vi "test_ParseSolutionFile.vi"() -> (3 "Pass?":bool)   [LabVIEW 2020, in "Tests.SolutionBuilder.lvlib"]
uses:
  Tests.SolutionBuilder.lvlib
  SolutionBuilder/SolutionBuilder.lvclass
panel:
  out "test results":u32 format="%03b"
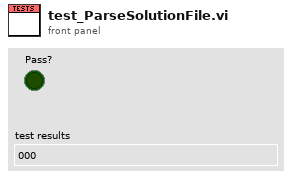
[diagram p1: front panel]
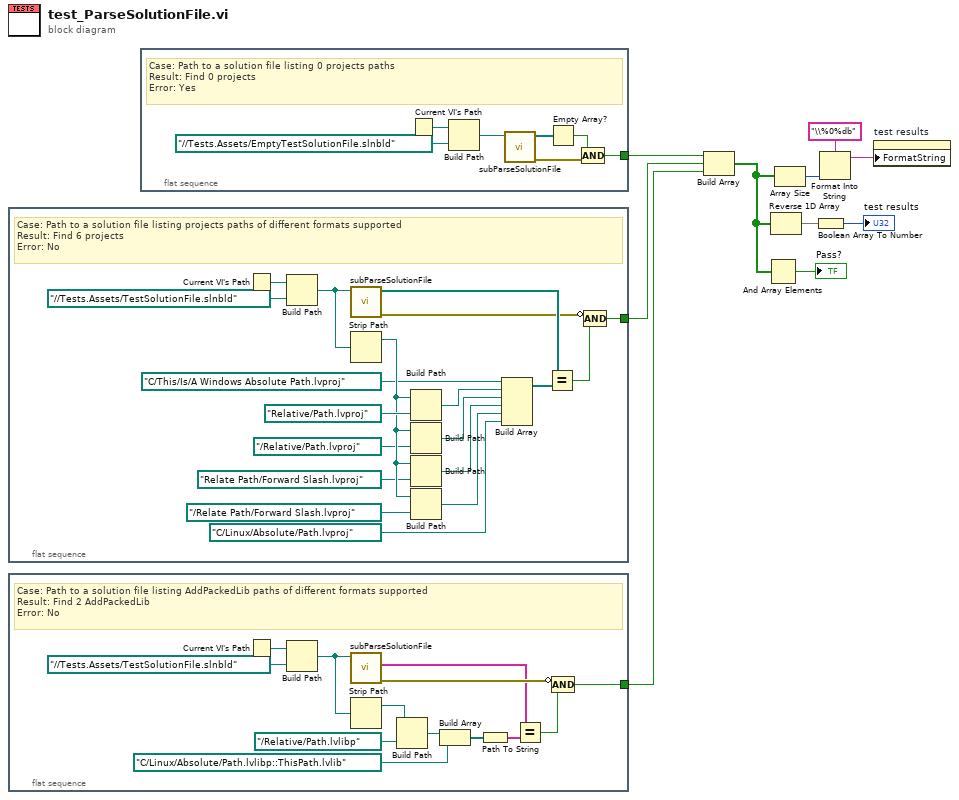
[diagram p0: block diagram]
diagram:
  n1 = flat-sequence {
    tunnel: [w11] -> w4
    frame #0 {
      # "Case: Path to a solution file listing projects paths of different formats supported\nResult: Find 6 projects\nError: No"
      n2 = Current VI's Path() -> (path=w29:path)
      n3 = Build Path(base path=w29, name or relative path=path "../../Tests.Assets/TestSolutionFile.slnbld" ("Path")) -> (appended path=w15:path)
      n4 = call "subParseSolutionFile.vi"("Solution file"=w15) -> ("error out"=w13:errorcluster, "Projects"=w14:path[])  [unwired: 8 in, 1 out]
      n5 = Strip Path(path=w15) -> (stripped path=w26:path)  [unwired: 1 out]
      n6 = Build Path(base path=w26, name or relative path=path "Relative/Path.lvproj" ("Path")) -> (appended path=w21:path)
      n7 = Build Path(base path=w26, name or relative path=path "../Relative/Path.lvproj" ("Path")) -> (appended path=w20:path)
      n8 = Build Path(base path=w26, name or relative path=path "Relate Path/Forward Slash.lvproj" ("Path")) -> (appended path=w19:path)
      n9 = Build Path(base path=w26, name or relative path=path "../Relate Path/Forward Slash.lvproj" ("Path")) -> (appended path=w18:path)
      n10 = Build Array(path "C:/This/Is/A Windows Absolute Path.lvproj" ("Path"), w21, w20, w19, w18, path "C:/Linux/Absolute/Path.lvproj" ("Path")) -> (w16:path[])
      n11 = Equal?(x=w14, y=w16) -> (x = y?=w12:bool)
      n12 = Compound Arithmetic op=AND(invert w13, w12) -> (w11:bool)
    }
  }
  n13 = flat-sequence {
    tunnel: [w33] -> w2
    frame #0 {
      # "Case: Path to a solution file listing AddPackedLib paths of different formats supported\nResult: Find 2 AddPackedLib\nError: No"
      n14 = Current VI's Path() -> (path=w42:path)
      n15 = Build Path(base path=w42, name or relative path=path "../../Tests.Assets/TestSolutionFile.slnbld" ("Path")) -> (appended path=w36:path)
      n16 = call "subParseSolutionFile.vi"("Solution file"=w36) -> ("error out"=w35:errorcluster, "Lib definition strings"=w32:string[])  [unwired: 8 in, 1 out]
      n17 = Strip Path(path=w36) -> (stripped path=w39:path)  [unwired: 1 out]
      n18 = Build Path(base path=w39, name or relative path=path "../Relative/Path.lvlibp" ("Path")) -> (appended path=w38:path)
      n19 = Build Array(w38, path "C:/Linux/Absolute/Path.lvlibp::ThisPath.lvlib" ("Path")) -> (w37:path[])
      n20 = Path To String(path=w37) -> (string=w31:string[])
      n21 = Equal?(x=w32, y=w31) -> (x = y?=w34:bool)
      n22 = Compound Arithmetic op=AND(invert w35, w34) -> (w33:bool)
    }
  }
  n23 = flat-sequence {
    tunnel: [w46] -> w3
    frame #0 {
      # "Case: Path to a solution file listing 0 projects paths\nResult: Find 0 projects\nError: Yes"
      n24 = Current VI's Path() -> (path=w47:path)
      n25 = Build Path(base path=w47, name or relative path=path "../../Tests.Assets/EmptyTestSolutionFile.slnbld" ("Path")) -> (appended path=w45:path)
      n26 = call "subParseSolutionFile.vi"("Solution file"=w45) -> ("error out"=w43:errorcluster, "Projects"=w44:path[])  [unwired: 8 in, 1 out]
      n27 = Empty Array?(array=w44) -> (empty?=w49:bool)
      n28 = Compound Arithmetic op=AND(w49, w43) -> (w46:bool)
    }
  }
  n29 = Build Array(w3, w4, w2) -> (w8:bool[])
  n30 = And Array Elements(Boolean array=w8) -> (logical AND=→"Pass?":bool)
  n31 = Reverse 1D Array(array=w8) -> (reversed array=w1:bool[])
  n32 = Array Size(array=w8) -> (size(s)=w6:i32)
  n33 = Boolean Array To Number(Boolean array=w1) -> (number=→"test results":u32)
  n34 = Format Into String(format string="\\%0%db", w6) -> (resulting string=w5:string)  [unwired: 2 in, 1 out]
  n35 = property on="test results" class="DigNum (strict)"("FormatString"=w5) -> ()  [unwired: 2 in, 2 out]
